vi "Channel Mng Update Test Cases.vi"() -> (0 "error out":errorcluster, 2 "status":string, 3 "pass":bool)   [LabVIEW 2021]
uses:
  Channels/CIFTag/Double/CIFTagDouble.lvclass
  D:/dev/CIF-LVCore/src/CIFUtilities/CIFChannels/CIFChannels.lvclass
  CIFChannels/Typedef/Direction.ctl
  CIFChannelMng.lvclass
  CIFChannels/CIFChannels.lvclass/CIFChannels.ctl
  CIFChannelMng.lvclass/CIFChannelMng.ctl
  CIFClocks/SubVIs/Add Error.vi
  CIFChannels/Accessors/Read Name.vi
  CIFChannels/Accessors/Read Custom Config Data.vi
  CIFChannels/Accessors/Read Channel Class.vi
  CIFChannels/Accessors/Read Direction.vi
  CIFCore/Common/Utilities/Append Error Location.vi
  CIFChannels/CIFChannels.lvclass
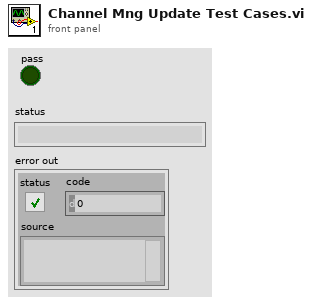
[diagram p1: front panel]
types:
  T1 = typedef "CIFChannels.lvclass/Direction.ctl" = enum16{"Publisher", "Subscriber"}
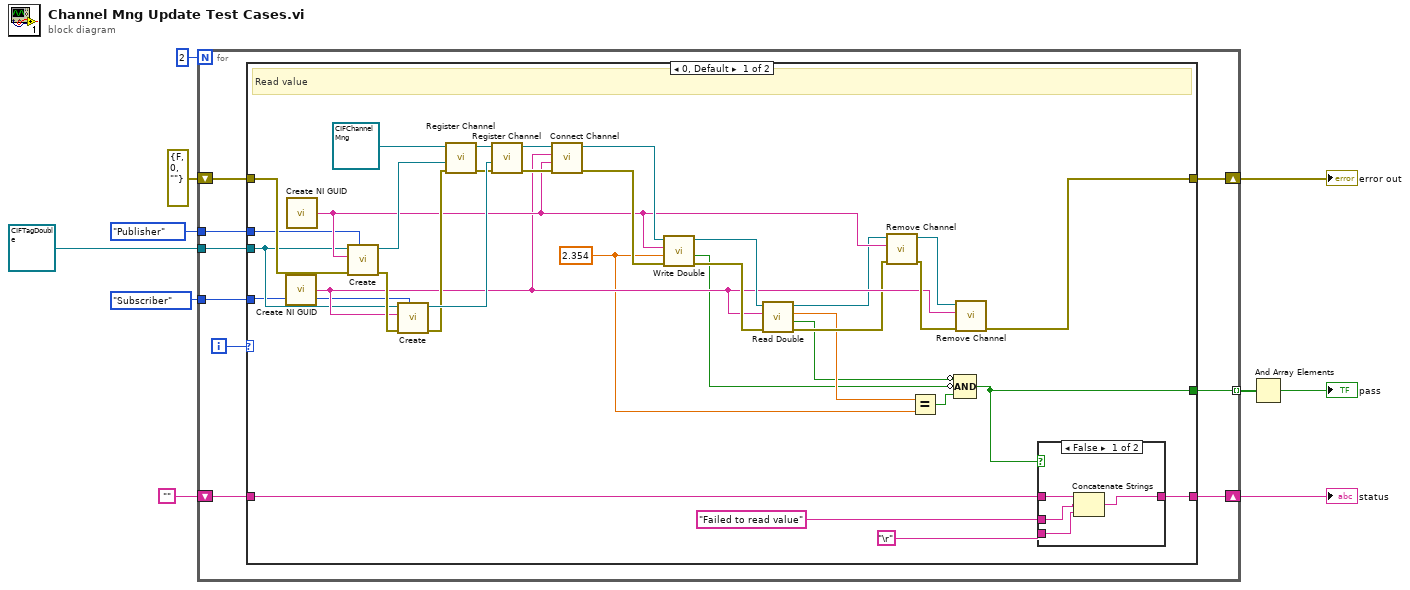
[diagram p0: block diagram]
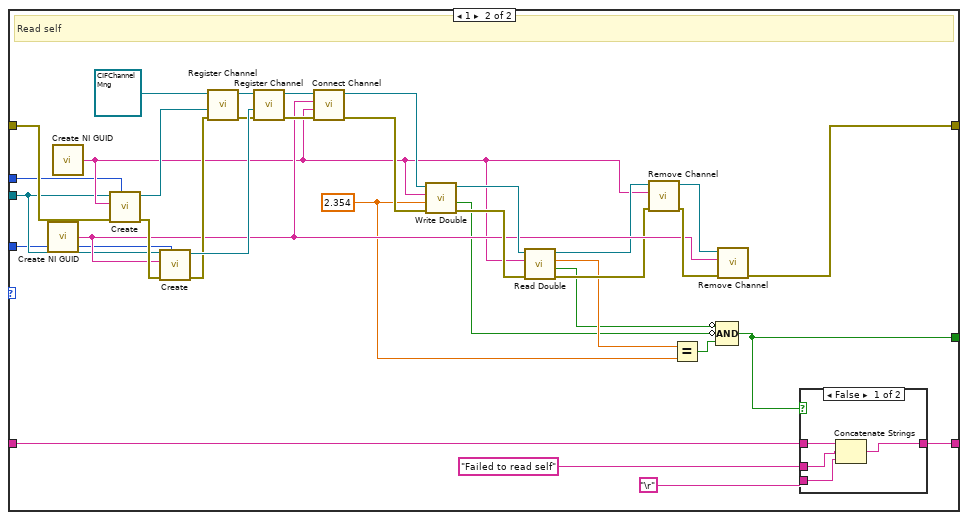
[diagram p3: hidden frame]
diagram:
  n1 = for {
    N: 2 -> [_]
    tunnel: [w19] -> w10 mode=indexing
    shift-right: [w17] -> w5
    shift-left: errorcluster {"status"=FALSE, "code"=0, "source"=""} ("error out") -> [w18]
    shift-right: [w14] -> w6
    shift-left: "" -> [w15]
    tunnel: refnum<class "CIFTagDouble.lvclass"> refnum ("CIFTagDouble.lvclass") -> [w13]
    tunnel: Direction."Subscriber" ("Direction") -> [w12]
    tunnel: Direction."Publisher" ("Direction") -> [w11]
    i -> [w16]
    n2 = case shown="0, Default" w16 {
      tunnel: [w48 w87] -> w19
      tunnel: w18 -> [w38 w77]
      tunnel: [w30 w70] -> w17
      tunnel: w15 -> [w53 w92]
      tunnel: [w52 w91] -> w14
      tunnel: w13 -> [w22 w61]
      tunnel: w12 -> [w21 w60]
      tunnel: w11 -> [w20 w59]
      frame 0, Default {
        w25 = 2.354
        # "Read value"
        n3 = call <vilib>:"Create NI GUID.vi"() -> ("NI GUID"=w29:string)
        n4 = call <vilib>:"Create NI GUID.vi"() -> ("NI GUID"=w33:string)
        n5 = call-dynamic "Create.vi"("Direction"=w20, "error in (no error)"=w38, "Name"=w33, "CIFTag in"=w22) -> ("error out"=w43:errorcluster, "CIFTag out"=w42:refnum<class "CIFTagDouble.lvclass">)  [unwired: 6 in]
        n6 = call-dynamic "Create.vi"("Direction"=w21, "error in (no error)"=w43, "Name"=w29, "CIFTag in"=w22) -> ("error out"=w44:errorcluster, "CIFTag out"=w47:refnum<class "CIFTagDouble.lvclass">)  [unwired: 6 in]
        n7 = call "Register Channel.vi"("error in (no error)"=w44, "Channel"=w42, "CIFChannelMng in"=refnum<class "CIFChannelMng.lvclass"> refnum) -> ("error out"=w41:errorcluster, "CIFChannelMng out"=w40:refnum<class "CIFChannelMng.lvclass">)  [unwired: 7 in]
        n8 = call "Register Channel.vi"("error in (no error)"=w41, "Channel"=w47, "CIFChannelMng in"=w40) -> ("error out"=w46:errorcluster, "CIFChannelMng out"=w45:refnum<class "CIFChannelMng.lvclass">)  [unwired: 7 in]
        n9 = call "Connect Channel.vi"("error in (no error)"=w46, "Publisher Name"=w33, "Subscriber Name"=w29, "CIFChannelMng in"=w45) -> ("error out"=w36:errorcluster, "CIFChannelMng out"=w37:refnum<class "CIFChannelMng.lvclass">)  [unwired: 6 in]
        n10 = call "Write Double.vi"("error in (no error)"=w36, "Data"=w25, "Channel Name"=w33, "CIFChannelMng in"=w37) -> ("error out"=w35:errorcluster, "timed out?"=w23:bool, "CIFChannelMng out"=w34:refnum<class "CIFChannelMng.lvclass">)  [unwired: 5 in]
        n11 = call "Read Double.vi"("error in (no error)"=w35, "Channel Name"=w29, "CIFChannelMng in"=w34) -> ("error out"=w28:errorcluster, "timed out?"=w24:bool, "Data"=w26:dbl, "CIFChannelMng out"=w27:refnum<class "CIFChannelMng.lvclass">)  [unwired: 5 in]
        n12 = call "Remove Channel.vi"("error in (no error)"=w28, "Channel Name"=w33, "CIFChannelMng in"=w27) -> ("error out"=w32:errorcluster, "CIFChannelMng out"=w31:refnum<class "CIFChannelMng.lvclass">)  [unwired: 7 in]
        n13 = Equal?(x=w26, y=w25) -> (x = y?=w49:bool)
        n14 = Compound Arithmetic op=AND(invert w24, invert w23, w49) -> (w48:bool)
        n15 = call "Remove Channel.vi"("error in (no error)"=w32, "Channel Name"=w29, "CIFChannelMng in"=w31) -> ("error out"=w30:errorcluster)  [unwired: 7 in, 1 out]
        n16 = case shown="False" w48 {
          tunnel: w53 -> [w57 w58]
          tunnel: [w54 w58] -> w52
          tunnel: "Failed to read value" -> [w56 _]
          tunnel: "\r" -> [w55 _]
          frame False {
            n17 = Concatenate Strings(w57, w56, w55) -> (w54:string)
          }
          frame True {
          }
        }
      }
      frame 1 {
        w65 = 2.354
        # "Read self"
        n18 = call <vilib>:"Create NI GUID.vi"() -> ("NI GUID"=w69:string)
        n19 = call <vilib>:"Create NI GUID.vi"() -> ("NI GUID"=w62:string)
        n20 = call-dynamic "Create.vi"("Direction"=w59, "error in (no error)"=w77, "Name"=w62, "CIFTag in"=w61) -> ("error out"=w82:errorcluster, "CIFTag out"=w81:refnum<class "CIFTagDouble.lvclass">)  [unwired: 6 in]
        n21 = call-dynamic "Create.vi"("Direction"=w60, "error in (no error)"=w82, "Name"=w69, "CIFTag in"=w61) -> ("error out"=w83:errorcluster, "CIFTag out"=w86:refnum<class "CIFTagDouble.lvclass">)  [unwired: 6 in]
        n22 = call "Register Channel.vi"("error in (no error)"=w83, "Channel"=w81, "CIFChannelMng in"=refnum<class "CIFChannelMng.lvclass"> refnum) -> ("error out"=w80:errorcluster, "CIFChannelMng out"=w79:refnum<class "CIFChannelMng.lvclass">)  [unwired: 7 in]
        n23 = call "Register Channel.vi"("error in (no error)"=w80, "Channel"=w86, "CIFChannelMng in"=w79) -> ("error out"=w85:errorcluster, "CIFChannelMng out"=w84:refnum<class "CIFChannelMng.lvclass">)  [unwired: 7 in]
        n24 = call "Connect Channel.vi"("error in (no error)"=w85, "Publisher Name"=w62, "Subscriber Name"=w69, "CIFChannelMng in"=w84) -> ("error out"=w75:errorcluster, "CIFChannelMng out"=w76:refnum<class "CIFChannelMng.lvclass">)  [unwired: 6 in]
        n25 = call "Write Double.vi"("error in (no error)"=w75, "Data"=w65, "Channel Name"=w62, "CIFChannelMng in"=w76) -> ("error out"=w74:errorcluster, "timed out?"=w63:bool, "CIFChannelMng out"=w73:refnum<class "CIFChannelMng.lvclass">)  [unwired: 5 in]
        n26 = call "Read Double.vi"("error in (no error)"=w74, "Channel Name"=w62, "CIFChannelMng in"=w73) -> ("error out"=w68:errorcluster, "timed out?"=w64:bool, "Data"=w66:dbl, "CIFChannelMng out"=w67:refnum<class "CIFChannelMng.lvclass">)  [unwired: 5 in]
        n27 = call "Remove Channel.vi"("error in (no error)"=w68, "Channel Name"=w62, "CIFChannelMng in"=w67) -> ("error out"=w72:errorcluster, "CIFChannelMng out"=w71:refnum<class "CIFChannelMng.lvclass">)  [unwired: 7 in]
        n28 = Equal?(x=w66, y=w65) -> (x = y?=w88:bool)
        n29 = Compound Arithmetic op=AND(invert w64, invert w63, w88) -> (w87:bool)
        n30 = call "Remove Channel.vi"("error in (no error)"=w72, "Channel Name"=w69, "CIFChannelMng in"=w71) -> ("error out"=w70:errorcluster)  [unwired: 7 in, 1 out]
        n31 = case shown="False" w87 {
          tunnel: w92 -> [w96 w97]
          tunnel: [w93 w97] -> w91
          tunnel: "Failed to read self" -> [w95 _]
          tunnel: "\r" -> [w94 _]
          frame False {
            n32 = Concatenate Strings(w96, w95, w94) -> (w93:string)
          }
          frame True {
          }
        }
      }
    }
  }
  "error out" <- w5
  "status" <- w6
  n33 = And Array Elements(Boolean array=w10) -> (logical AND=→"pass":bool)
